vi "TrackerMain.vi"(11 "MeasureConfig":T1={"Bead locations"=[{"X"=0, "Y"=0}], "ROI"=200, "Experiment base path"=path "", "Image output subdir"="images", "Output mode"=enum."None", "Traces output subdir"="traces", "QTrk Settings"={"Image width"=150, "Image height"=150, "Number of threads (CPU based)"=-1, "CUDA Device"=-2, "COM Background correction factor"=0.0, "ZLUT MinRadius"=8.0, "ZLUT Radial sample density"=5.0, "ZLUT Angular sample density"=2.0, "ZLUT ROI Coverage"=0.7, "QI Iterations"=1, "QI MinRadius"=2.0, "QI Radial sample density"=5.0, "QI Angular sample density"=2.0, "QI ROI Coverage"=0.7, "QI Angular Step \nIteration Factor"=0.8, "XCOR Profile Length"=1, "XCOR Profile Width"=128, "XCOR Iterations"=32, "Gaussian 2D Fit Iterations"=2, "Gaussian 2D Sigma (pixels)"=3.0, "Downsample"=0}, "Tracking Config"={"Number of steps"=0, "ZLUT stepsize (um)"=0.0, "Z correction factor"=0.0, "Start piezo Z (um)"=0.0, "Pixel size (nm)"=0.0, "2D Localization Type"=enum."Quadrant Interpolation", "Z Command (None)"=enum."Nothing", "Z Piezo scale"=FALSE, "ZLUT Building\nimages per frame"=0, "ZLUT Bias correction planes"=1}, "Experiment Name"="", "Program"={"Commands"=[], "Motor Axis accuracy conditions"={"Magnet Z"=0.0, "Magnet rotation"=0.0, "Camera"={"X"=0.0, "Y"=0.0}, "Piezo XY"={"X"=0.0, "Y"=0.0}, "Piezo Z"=0.0}, "Axis flags"={"Magnet Z"=FALSE, "Magnet rotation"=FALSE, "Camera"={"X"=FALSE, "Y"=FALSE}, "Piezo XY"={"X"=FALSE, "Y"=FALSE}, "Piezo Z"=FALSE}}, "ZLUT"=[], "Camera settings"={"Framerate (Hz)"=60, "Exposure time (us)"=5000, "Image size"={"Width"=1280, "Height"=1024}, "Number of buffers"=30}, "Experiment Script"="", "Max frames in memory"=10000, "Save traces as binary"=FALSE, "Pixel Calibration Gain Image"="camera_calib_gain.bin", "Pixel Calibration Offset Image"="camera_calib_offset.bin", "Use pixel calibration images"=FALSE, "Internal camera settings"="", "Trace write interval"=100, "ExperimentComment"=""} {"QTrk Settings"."QI ROI Coverage" format="%_2g"; "QTrk Settings"."QI MinRadius" format="%.2f"; "QTrk Settings"."QI Angular sample density" format="%.3f"; "QTrk Settings"."QI Radial sample density" format="%.2f"; "QTrk Settings"."ZLUT Radial sample density" format="%.2f"; "QTrk Settings"."ZLUT MinRadius" format="%.2f"}) -> (0 "Section list":i32[](array[numeric]))   [LabVIEW 2011]
uses:
  Typedefs/MeasureConfigType.ctl
  Typedefs/MeasureConfigOutputMode.ctl
  qtrk/QTrkLVBinding/QTrkSettings.ctl
  Typedefs/TrackingConfigType.ctl
  qtrk/QTrkLVBinding/QTrkLocalizationType.ctl
  qtrk/QTrkLVBinding/QTrkZCommandType.ctl
  ExperimentProgram/ExperimentProgramType.ctl
  ExperimentProgram/ExProgCommandType.ctl
  ExperimentProgram/ExProgCommandEnumType.ctl
  Motors/MotorAxisEnum.ctl
  Motors/MotorPosType.ctl
  Typedefs/XYf.ctl
  Motors/MotorPosFlagsType.ctl
  Camera/GenericCameraConfigType.ctl
  Typedefs/CmdEnum_UserInterfaceCmd.ctl
  qtrk/QTrkLVBinding/ResultManagerConfig.ctl
  qtrk/QTrkLVBinding/XYZf.ctl
  Camera/CIGrabParams.ctl
  qtrk/QTrkLVBinding/QTrkInstance.ctl
  qtrk/QTrkLVBinding/ResultManagerInstance.ctl
  Camera/CIGrabControlMsg.ctl
  Camera/CIGrabControlMsgEnum.ctl
  GlobalVariables.vi
panel:
  out "ZLUT Correction":sgl[][](graph)
  out "Lost frames":i32
  in  "Offset factor":dbl=1.0
  in  "Gain factor":dbl=1.0
  in  "Close dialog":bool
  out "Framerate":i32
  out "Localizations done":i32
  out "Captured frames":i32
  out "Tracker internal profiling info":string
  out "Tracking queue %":i32
  out "[base]\\traces\\[expname].txt":path
  out "[base]\\traces\\[expname]_motors.txt":path
  out "Saved frames":i32
  out "Time (s)":dbl
  out "Script Complete":bool
  out "Instruction index":i32
  in  "End experiment":bool
  out "Frames complete":i32
  # "Running experiment"
  # "(used for commands with string parameters)"
  # "-2: Use all devices\n-1: Use best device"
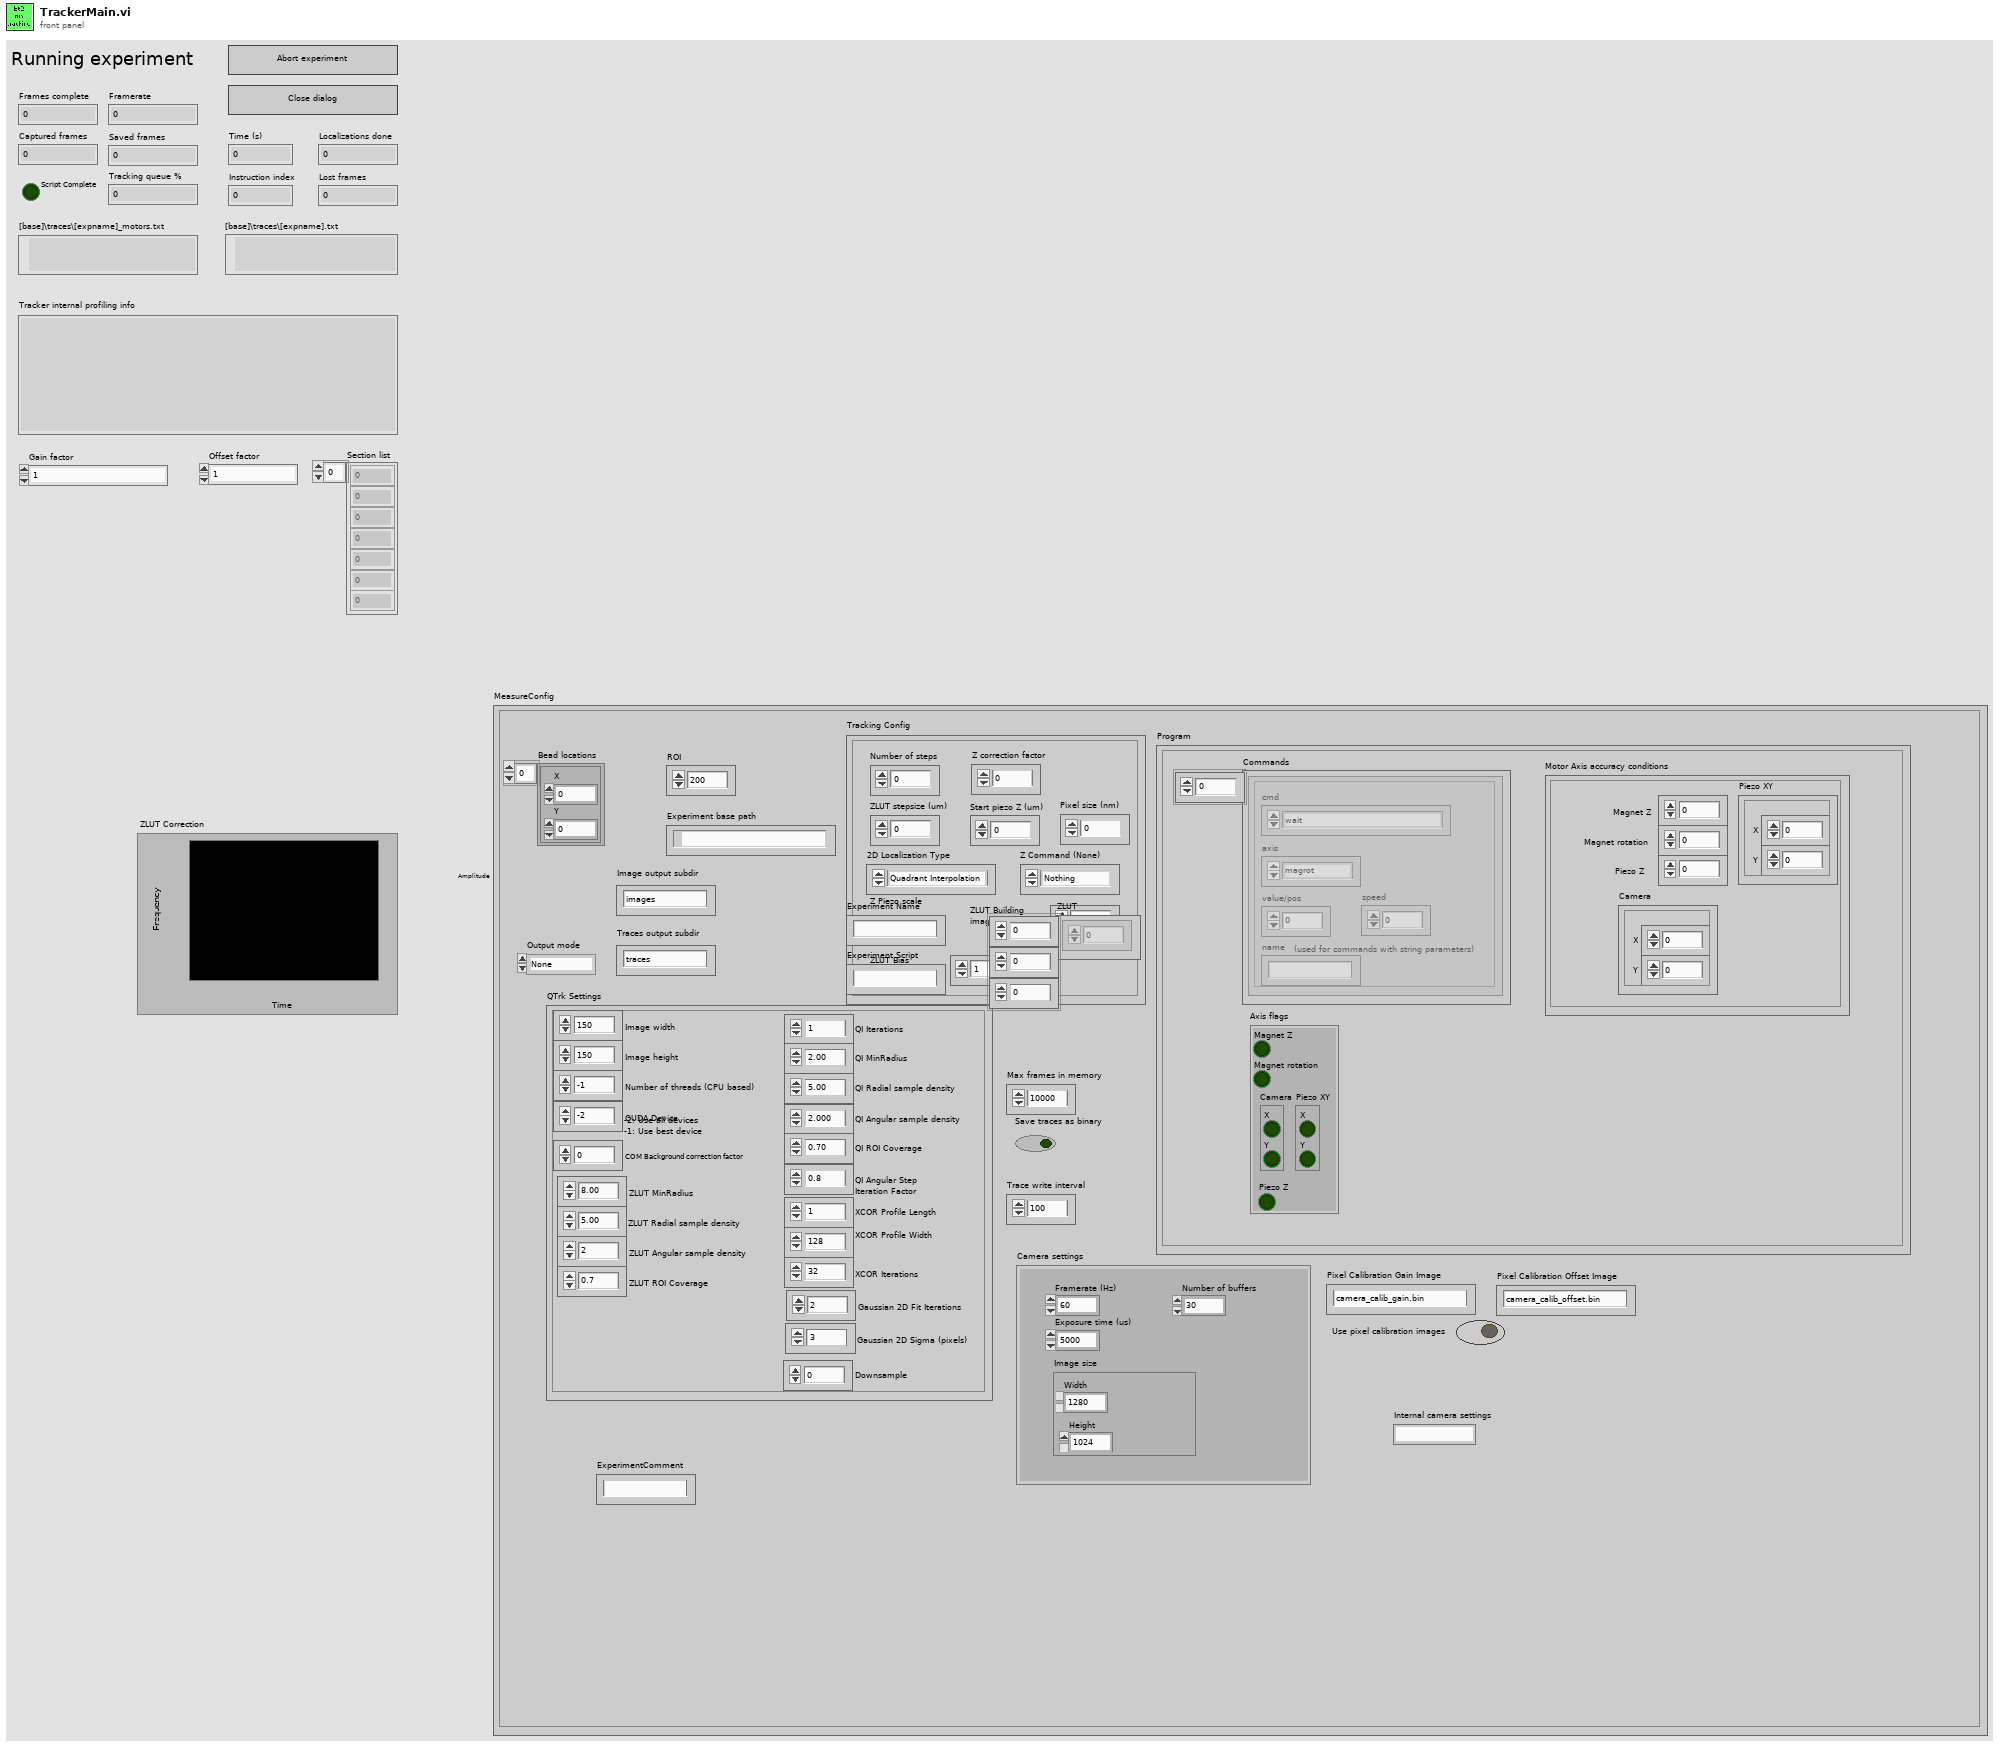
[diagram p1: front panel]
types:
  T1 = typedef "MeasureConfigType.ctl" = cluster{"Bead locations":cluster{"X":i32, "Y":i32}[], "ROI":i32, "Experiment base path":path, "Image output subdir":string, "Output mode":T2, "Traces output subdir":string, "QTrk Settings":T3, "Tracking Config":T4, "Experiment Name":string, "Program":T7, "ZLUT":sgl[][][], "Camera settings":T14, "Experiment Script":string, "Max frames in memory":i32, "Save traces as binary":bool, "Pixel Calibration Gain Image":string, "Pixel Calibration Offset Image":string, "Use pixel calibration images":bool, "Internal camera settings":string, "Trace write interval":i32, "ExperimentComment":string}
  T2 = typedef "MeasureConfigOutputMode.ctl" = enum16{"None", "Track", "SaveImages"}
  T3 = typedef "QTrkSettings.ctl" = cluster{"Image width":i32, "Image height":i32, "Number of threads (CPU based)":i32, "CUDA Device":i32, "COM Background correction factor":sgl, "ZLUT MinRadius":sgl, "ZLUT Radial sample density":sgl, "ZLUT Angular sample density":sgl, "ZLUT ROI Coverage":sgl, "QI Iterations":i32, "QI MinRadius":sgl, "QI Radial sample density":sgl, "QI Angular sample density":sgl, "QI ROI Coverage":sgl, "QI Angular Step \nIteration Factor":sgl, "XCOR Profile Length":i32, "XCOR Profile Width":i32, "XCOR Iterations":i32, "Gaussian 2D Fit Iterations":i32, "Gaussian 2D Sigma (pixels)":sgl, "Downsample":i32}
  T4 = typedef "TrackingConfigType.ctl" = cluster{"Number of steps":i32, "ZLUT stepsize (um)":sgl, "Z correction factor":sgl, "Start piezo Z (um)":sgl, "Pixel size (nm)":sgl, "2D Localization Type":T5, "Z Command (None)":T6, "Z Piezo scale":bool, "ZLUT Building\nimages per frame":i32, "ZLUT Bias correction planes":i32}
  T5 = typedef "QTrkLocalizationType.ctl" = enum16{"Center-of-Mass", "1D Cross-Correlation", "Quadrant Interpolation", "Gaussian 2D MLE", "QI + ZLUTAlign", "ZLUTAlign", "QI + FourierLUT"}
  T6 = typedef "QTrkZCommandType.ctl" = enum16{"Nothing", "ComputeZ", "BuildRadialZLUT", "BuildImageZLUT", "RadialZLUT+ImageZLUT"}
  T7 = typedef "ExperimentProgramType.ctl" = cluster{"Commands":T8[], "Motor Axis accuracy conditions":T11, "Axis flags":T13}
  T8 = typedef "ExProgCommandType.ctl" = cluster{"cmd":T9, "axis":T10, "value/pos":dbl, "speed":dbl, "name":string}
  T9 = typedef "ExProgCommandEnumType.ctl" = enum16{"wait", "move", "event", "idle", "when", "section", "stop"}
  T10 = typedef "MotorAxisEnum.ctl" = enum16{"no axis", "magrot", "magpos", "px", "py", "pz", "camx", "camy"}
  T11 = typedef "MotorPosType.ctl" = cluster{"Magnet Z":dbl, "Magnet rotation":dbl, "Camera":T12, "Piezo XY":T12, "Piezo Z":dbl}
  T12 = typedef "XYf.ctl" = cluster{"X":sgl, "Y":sgl}
  T13 = typedef "MotorPosFlagsType.ctl" = cluster{"Magnet Z":bool, "Magnet rotation":bool, "Camera":cluster{"X":bool, "Y":bool}, "Piezo XY":cluster{"X":bool, "Y":bool}, "Piezo Z":bool}
  T14 = typedef "GenericCameraConfigType.ctl" = cluster{"Framerate (Hz)":i32, "Exposure time (us)":i32, "Image size":cluster{"Width":i32, "Height":i32}, "Number of buffers":i32}
  T15 = typedef "CmdEnum_UserInterfaceCmd.ctl" = enum32{"Idle (Use for default)", "ResultTracesUpdated", "MeasureConfigUpdated", "MeasureEnd", "MeasureStart"}
  T16 = typedef "ResultManagerConfig.ctl" = cluster{"Number of beads":i32, "Number of frame info columns":i32, "Result scaling":T17, "Result offset":T17, "Write Interval":i32, "Max frames in memory":i32, "Binary output (1/0)":i8}
  T17 = typedef "XYZf.ctl" = cluster{"X":sgl, "Y":sgl, "Z":sgl}
  T18 = typedef "ResultManagerInstance.ctl" = cluster{"InstancePtr":u64}
  T19 = typedef "QTrkInstance.ctl" = cluster{"QTrk Pointer":u64}
  T20 = typedef "CIGrabParams.ctl" = cluster{"QTrk Instance":T19, "ResultManager":T18, "Send to queue?":bool, "Force full-frame capture":bool}
  T21 = typedef "CIGrabControlMsg.ctl" = cluster{"Msg":T22}
  T22 = typedef "CIGrabControlMsgEnum.ctl" = enum16{"Stop", "EnableTracking", "DisableTracking"}
  T23 = typedef "PixelCalibrationDataType.ctl" = cluster{"Offset image":T24, "Gain image":T24, "Use offset":bool, "Use gain":bool}
  T24 = typedef "IMAQ Image.ctl" = refnum<image>
  T25 = typedef "CameraInstance.ctl" = cluster{"VI refs":T26, "Camera state":variant}
  T26 = typedef "CameraInterface.ctl" = cluster{"Close":T27, "Get/Set generic config":T28, "Grab":T29, "Show Settings Dialog":T30, "AdjustBeadPos":T31, "Save/load camera settings":T32}
  T27 = typedef "CICloseType.ctl" = refnum<vi>
  T28 = typedef "CIGetSetGenericConfig.ctl" = refnum<vi>
  T29 = typedef "CIGrabType.ctl" = refnum<vi>
  T30 = typedef "CISettingsDlg.ctl" = refnum<vi>
  T31 = typedef "CIAdjustBeadPos.ctl" = refnum<vi>
  T32 = typedef "CISaveLoadSettings.ctl" = refnum<vi>
  T33 = typedef "ExProgState.ctl" = cluster{"Wanted Motorpos":T11, "Goal motorpos":T11, "Instruction":i32, "Speed":T11, "New instruction?":bool, "Instruction start time":dbl}
  T34 = typedef "QueueListType.ctl" = cluster{"Motor In":refnum<queue>, "User Interface Image View":refnum<queue>, "User Interface Camera Control":refnum<queue>, "User Interface Event Notifier":refnum<notifier>, "Initialized?":bool, "Experiment Script Event Notifier":refnum<notifier>}
  T35 = cluster{"Script loop delay":i32, "Motor loop ":i32, "Motor get pos wait time\nper axis":i32}
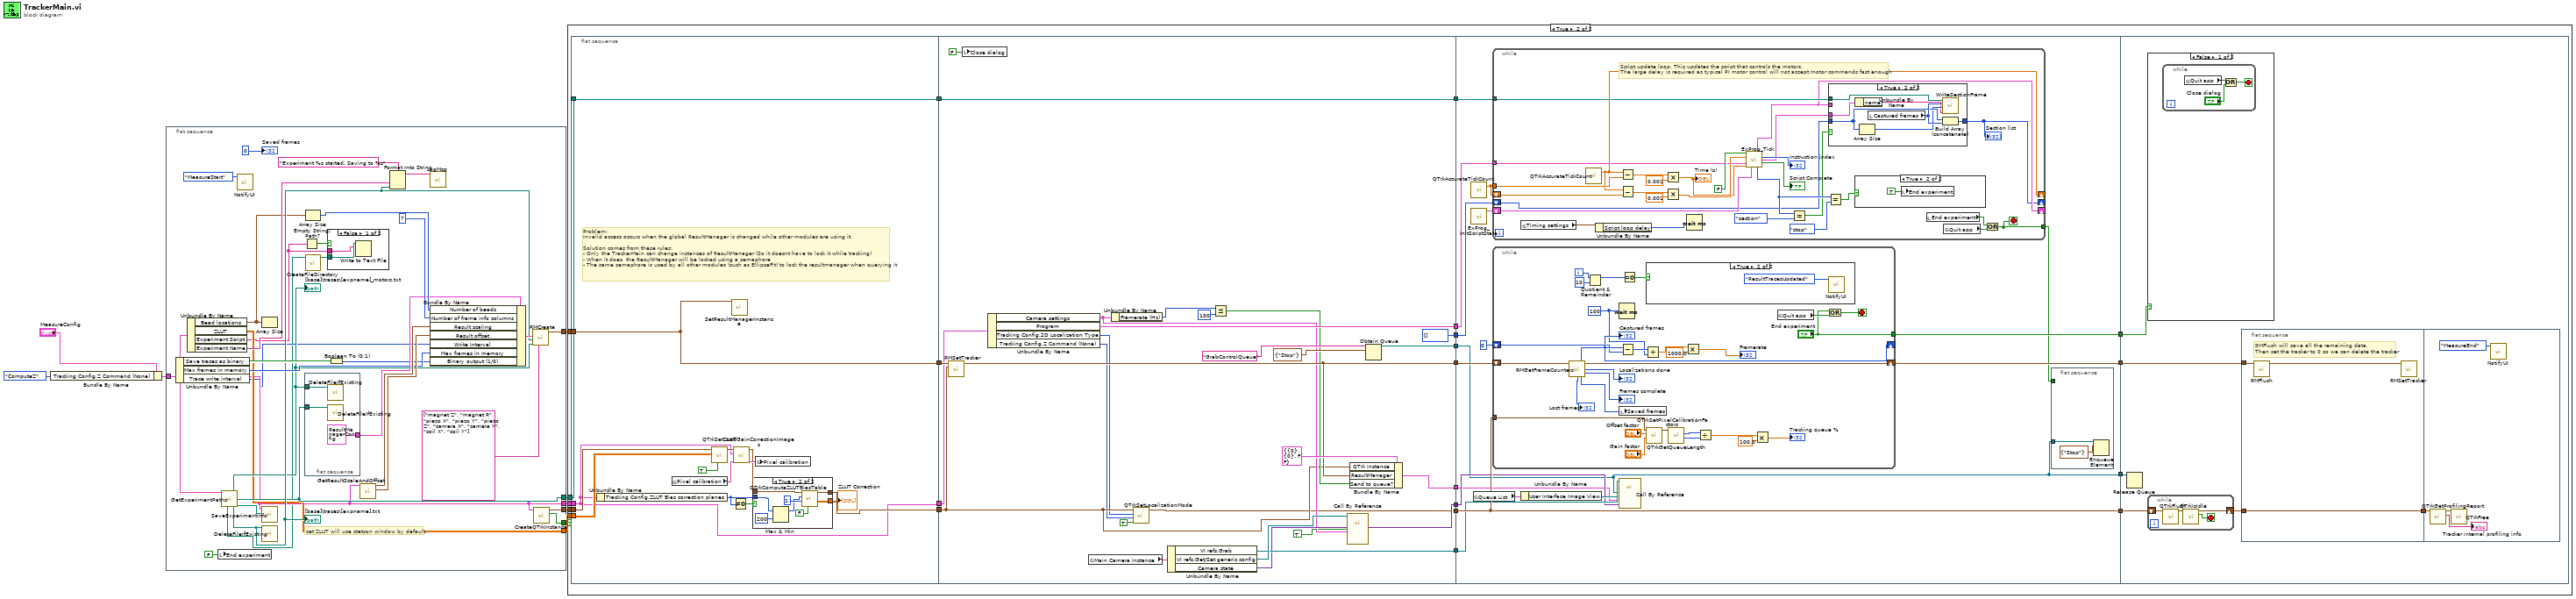
[diagram p0: block diagram]
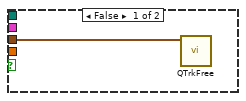
[diagram p2: hidden frame]
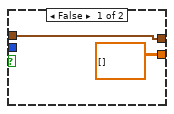
[diagram p3: hidden frame]
diagram:
  n1 = Bundle By Name(cluster="MeasureConfig", "Tracking Config.Z Command (None)"=QTrkZCommandType."ComputeZ") -> (w2:T1)
  n2 = flat-sequence {
    tunnel: [w19] -> w9
    tunnel: [w22] -> w7
    tunnel: [w21] -> w8
    tunnel: [w20] -> w6
    tunnel: [w16] -> w5
    tunnel: [w18] -> w4
    tunnel: w2 -> [w16]
    frame #0 {
      # "set ZLUT will use stetson window by default"
      n3 = Unbundle By Name(w16) -> ("Save traces as binary"=w29:bool, "Max frames in memory"=w30:i32, "Trace write interval"=w11:i32)
      n4 = Unbundle By Name(w16) -> ("Bead locations"=w17:cluster{"X":i32, "Y":i32}[], "ZLUT"=w20:sgl[][][], "Experiment Script"=w15:string, "Experiment Name"=w26:string)
      n5 = local write "End experiment"(FALSE ("End experiment")) -> ()
      n6 = call "GetExperimentPaths.vi"("MeasureConfig"=w16) -> ("[base]\\traces\\[expname]_motors.txt"=w23:path, "[base]\\traces\\[expname]_sections.txt"=w22:path, "[base]\\[expname]_script.txt"=w10:path, "[base]\\traces\\[expname].txt/bin"=w25:path, "[base]\\traces\\[expname]_info.txt"=w39:path)  [unwired: 6 in, 4 out]
      "[base]\\traces\\[expname]_motors.txt" <- w23
      "[base]\\traces\\[expname].txt" <- w25
      n7 = call "NotifyUI.vi"("User Interface Commands"=CmdEnum_UserInterfaceCmd."MeasureStart") -> ()  [unwired: 11 in]
      n8 = Array Size(array=w17) -> ()  [unwired: 1 out]
      n9 = call "SaveExperimentInfo.vi"("Filename"=w39, "MeasureConfig"=w16) -> ()  [unwired: 10 in]
      n10 = call "DeleteFileIfExisting.vi"("filename"=w25) -> ()  [unwired: 11 in]
      n11 = Empty String/Path?(string/path=w15) -> (empty?=w14:bool)
      n12 = flat-sequence {
        tunnel: [T16 {"Number of beads"=0, "Number of frame info columns"=0, "Result scaling"={"X"=0.0, "Y"=0.0, "Z"=0.0}, "Result offset"={"X"=0.0, "Y"=0.0, "Z"=0.0}, "Write Interval"=0, "Max frames in memory"=0, "Binary output (1/0)"=0} ("ResultManagerConfig")] -> w31
        tunnel: w23 -> [w44]
        tunnel: w22 -> [w43]
        frame #0 {
          n13 = call "DeleteFileIfExisting.vi"("filename"=w44) -> ()  [unwired: 11 in]
          n14 = call "DeleteFileIfExisting.vi"("filename"=w43) -> ()  [unwired: 11 in]
        }
      }
      n15 = Array Size(array=w17) -> (size(s)=w32:i32)
      n16 = call "CreateFileDirectory.vi"("filename"=w10) -> ("filename (copy)"=w38:path)  [unwired: 10 in]
      n17 = case shown="False" w14 {
        tunnel: w38 -> [w42 _]
        tunnel: w15 -> [w41 _]
        frame False {
          n18 = Write to Text File(file (use dialog)=w42, text=w41) -> ()  [unwired: 2 in, 3 out]
        }
        frame True {
        }
      }
      n19 = Boolean To (0,1)(Boolean=w29) -> (0, 1=w28:i16)
      n20 = call "GetResultScaleAndOffset.vi"("MeasureConfig"=w16) -> ("offset"=w33:cluster{dbl, dbl, "y":sgl}, "scale"=w34:cluster{sgl, sgl, sgl})  [unwired: 9 in]
      n21 = Format Into String(format string="Experiment %s started. Saving to %s", w26, w25) -> (resulting string=w24:string)  [unwired: 2 in, 1 out]
      n22 = call "LogMsg.vi"("msg"=w24) -> ()  [unwired: 11 in]
      n23 = Bundle By Name(cluster=w31, "Number of beads"=w32, "Number of frame info columns"=7, "Result scaling"=w34, "Result offset"=w33, "Write Interval"=w11, "Max frames in memory"=w30, "Binary output (1/0)"=w28) -> (w36:T16)
      n24 = call "RMCreate.vi"("Frame info names"=string[] ["magnet Z", "magnet R", "piezo X", "piezo Y", "piezo Z", "camera X", "camera Y", "coil X", "coil Y"], "frame info file"=w23, "output file"=w25, "ResultManagerConfig"=w36) -> ("ResultManager"=w21:T18)  [unwired: 7 in]
      n25 = call "CreateQTrkInstance.vi"("MeasureConfig"=w16) -> ("Go-ahead?"=w18:bool, "QTrk Instance"=w19:T19)  [unwired: 9 in]
      "Saved frames" <- 0 ("Saved frames")
    }
  }
  n26 = case shown="True" w4 {
    tunnel: w9 -> [w46 w60]
    tunnel: w8 -> [_ w59]
    tunnel: w7 -> [_ w58]
    tunnel: w6 -> [_ w57]
    tunnel: w5 -> [_ w56]
    frame False {
      n27 = call "QTrkFree.vi"("QTrk Instance"=w46) -> ()  [unwired: 6 in, 1 out]
    }
    frame True {
      n28 = flat-sequence {
        tunnel: [w79] -> w68
        tunnel: [w82] -> w67
        tunnel: w60 -> [w81]
        tunnel: w59 -> [w79]
        tunnel: w58 -> [w82]
        tunnel: w57 -> [w74]
        tunnel: w56 -> [w69]
        tunnel: [w69] -> w55
        tunnel: [w75] -> w47
        tunnel: [w115] -> w66
        tunnel: w68 -> [w119]
        tunnel: [w105] -> w65
        tunnel: [w96] -> w64
        tunnel: [i32[] [] ("initialized array")] -> w63
        tunnel: w67 -> [w117]
        tunnel: [w117] -> w62
        tunnel: [w104] -> w61
        tunnel: w55 -> [w116]
        tunnel: [w109] -> w51
        tunnel: [w107] -> w49
        tunnel: [w103] -> w48
        tunnel: w47 -> [w97]
        tunnel: w66 -> [w135]
        tunnel: w65 -> [w133]
        tunnel: w64 -> [w127]
        tunnel: w63 -> [w132]
        tunnel: w62 -> [w131]
        tunnel: w61 -> [w120]
        tunnel: [w129] -> w54
        tunnel: [w128] -> w53
        tunnel: [w127] -> w52
        tunnel: w51 -> [w126]
        tunnel: [w121] -> w50
        tunnel: w49 -> [w122]
        tunnel: w48 -> [w121]
        tunnel: w54 -> [w208]
        tunnel: w53 -> [w212]
        tunnel: w52 -> [w211]
        tunnel: w50 -> [w207]
        frame #0 {
          # "Problem: \nInvalid access occurs when the global ResultManager is changed while other modules are using it.\n\nSolution comes from these rules:\n- Only the TrackerMain can change instances of ResultManager (So it doesnt have to lock it while tracking)\n- When it does, the ResultManager will be locked using a semaphore\n- The same semaphore is used by all other modules (such as EllipseFit) to lock the resultmanager when querying it"
          n29 = Unbundle By Name(w69) -> ("Tracking Config.ZLUT Bias correction planes"=w70:i32)
          n30 = global read "GlobalVariables.vi" "Pixel calibration"() -> (w78:T23)
          n31 = call "QTrkSetZLUT.vi"("Normalize LUT"=TRUE, "ZLUT"=w74, "QTrk Instance"=w81) -> ("QTrk Instance"=w80:T19)  [unwired: 7 in, 1 out]
          n32 = call "SetResultManagerInstance.vi"("ResultManager"=w79) -> ()  [unwired: 11 in]
          n33 = Not Equal To 0?(x=w70) -> (x != 0?=w71:bool)
          n34 = call "LoadGainCorrectionImages.vi"("Pixel calibration"=w78, "MeasureConfig"=w69, "QTrk Instance in"=w80) -> ("Pixel calibration(out)"=w77:T23, "QTrk Instance out"=w76:T19)  [unwired: 7 in]
          n35 = case shown="True" w71 {
            tunnel: w76 -> [w84 w92]
            tunnel: [w84 w91] -> w75
            tunnel: [sgl[][] [] ("Bias correction table") w88] -> w73
            tunnel: w70 -> [_ w85]
            frame False {
            }
            frame True {
              n36 = Max & Min(x=w85, y=200) -> (max(x,y)=w86:i32)  [unwired: 1 out]
              n37 = call "QTrkComputeZLUTBiasTable.vi"("Use spline interpolation?"=FALSE, "smpPerPixel"=1, "bias planes"=w86, "QTrk Instance"=w92) -> ("Bias correction table"=w88:sgl[][], "QTrk Instance"=w91:T19)  [unwired: 5 in, 1 out]
            }
          }
          "ZLUT Correction" <- w73
          n38 = global write "GlobalVariables.vi" "Pixel calibration"(w77) -> ()
        }
        frame #1 {
          n39 = call "RMSetTracker.vi"("QTrk Instance"=w97, "ResultManager"=w119) -> ("ResultManager (out)"=w105:T18)  [unwired: 8 in, 1 out]
          n40 = local write "Close dialog"(FALSE ("Close dialog")) -> ()
          n41 = Unbundle By Name(w116) -> ("Camera settings"=w102:T14, "Program"=w115:T7, "Tracking Config.2D Localization Type"=w95:T5, "Tracking Config.Z Command (None)"=w94:T6)
          n42 = global read "GlobalVariables.vi" "Main Camera Instance"() -> (w111:T25)
          n43 = Unbundle By Name(w102) -> ("Framerate (Hz)"=w101:i32)
          n44 = call "QTrkSetLocalizationMode.vi"("Normalize profile"=TRUE, "Z Command"=w94, "2D Localization Type"=w95, "QTrk Instance"=w97) -> ("QTrk Instance"=w96:T19)  [unwired: 7 in]
          n45 = Unbundle By Name(w111) -> ("VI refs.Grab"=w109:T29, "VI refs.Get/Set generic config"=w110:T28, "Camera state"=w108:variant)
          n46 = Less Or Equal?(x=w101, y=100 ("x")) -> (x <= y?=w99:bool)
          n47 = call-by-ref "?"(reference=w110, "Set? (F)"=TRUE, "GenericCameraConfig"=w102, "Camera state"=w108) -> ("Camera state (out)"=w107:variant)  [unwired: 8 in, 3 out]
          n48 = Bundle By Name(cluster=T20 {"QTrk Instance"={"QTrk Pointer"=0}, "ResultManager"={"InstancePtr"=0}, "Send to queue?"=FALSE, "Force full-frame capture"=FALSE} ("TrackingParameters"), "QTrk Instance"=w97, "ResultManager"=w105, "Send to queue?"=w99) -> (w104:T20)
          n49 = Obtain Queue(name (unnamed)="GrabControlQueue", element data type=T21 {"Msg"=enum."Stop"} ("GrabControlMsg")) -> (queue out=w103:refnum<queue>)  [unwired: 3 in, 2 out]
        }
        frame #2 {
          n50 = call "QTrkAccurateTickCount.vi"() -> ("tick count (ms)"=w134:dbl)  [unwired: 2 in, 1 out]
          n51 = call "ExProg_InitScriptState.vi"() -> ("Script exec state out"=w136:T33)  [unwired: 11 in]
          n52 = global read "GlobalVariables.vi" "Queue List"() -> (w124:T34)
          n53 = while {
            shift-right: [w175] -> _
            shift-left: w136 -> [w193]
            shift-right: [w190] -> _
            shift-left: w134 -> [w194]
            tunnel: w135 -> [w174]
            tunnel: w134 -> [w189]
            shift-right: [w173] -> _
            shift-left: w132 -> [w177]
            tunnel: w131 -> [w176]
            tunnel: [w171] -> w125
            stop <- w171 stop-if-true
            # "Script update loop. This updates the script that controls the motors.\nThe large delay is required as typical PI motor control will not accept motor commands fast enough"
            n54 = global read "GlobalVariables.vi" "Timing settings"() -> (w170:T35)
            n55 = call "QTrkAccurateTickCount.vi"() -> ("tick count (ms)"=w190:dbl)  [unwired: 2 in, 1 out]
            n56 = Unbundle By Name(w170) -> ("Script loop delay"=w169:i32)
            n57 = Subtract(x=w190, y=w189) -> (x-y=w188:dbl)
            n58 = Subtract(x=w190, y=w194) -> (x-y=w185:dbl)
            n59 = Multiply(x=w188, y=0.001) -> (x*y=w183:dbl)
            "Time (s)" <- w183
            n60 = Multiply(x=w185, y=0.001) -> (x*y=w184:dbl)
            n61 = Wait (ms)(milliseconds to wait=w169) -> ()  [unwired: 1 out]
            n62 = call "ExProg_Tick.vi"("Simulation?"=FALSE, "Timestep (s)"=w184, "Program"=w174, "Current time (s)"=w183, "Script exec state in"=w193) -> ("Script exec state out"=w175:T33, "Instruction index"=→"Instruction index":i32, "Last instruction"=w172:T8, "script ended?"=→"Script Complete":bool, "Last command"=w180:T9)  [unwired: 6 in]
            n63 = Equal?(x=w180, y=ExProgCommandEnumType."section") -> (x = y?=w178:bool)
            n64 = Equal?(x=w180, y=ExProgCommandEnumType."stop") -> (x = y?=w181:bool)
            n65 = case shown="True" w178 {
              tunnel: w177 -> [w198 w202]
              tunnel: [w198 w205] -> w173
              tunnel: w176 -> [_ w204]
              tunnel: w175 -> [_ _]
              tunnel: w172 -> [_ w199]
              frame False {
              }
              frame True {
                n66 = Unbundle By Name(w199) -> ("name"=w200:string)
                n67 = Array Size(array=w202) -> (size(s)=w201:i32)
                n68 = local read "Captured frames"() -> (w203:i32)
                n69 = call "WriteSectionFrame.vi"("section name"=w200, "section index"=w201, "section frame"=w203, "[base]\\traces\\[expname]_sections.txt"=w204) -> ()  [unwired: 8 in]
                n70 = Build Array (concatenate)(w202, w203) -> (w205:i32[])
              }
            }
            "Section list" <- w173
            n71 = case shown="True" w181 {
              frame False {
              }
              frame True {
                n72 = local write "End experiment"(TRUE ("End experiment")) -> ()
              }
            }
            n73 = local read "End experiment"() -> (w197:bool)
            n74 = global read "GlobalVariables.vi" "Quit app"() -> (w196:bool)
            n75 = Or(x=w197, y=w196) -> (x .or. y?=w171:bool)
          }
          n76 = while {
            tunnel: ["End experiment"] -> w128
            tunnel: w127 -> [w143]
            shift-right: [w164] -> w129
            shift-left: w133 -> [w163]
            shift-right: [w150] -> _
            shift-left: 0 ("capturedFrames") -> [w149]
            i -> [w160]
            stop <- w166 stop-if-true
            w147 = u32 100 ("milliseconds to wait")
            n77 = call "RMGetFrameCounters.vi"("ResultManager"=w163) -> ("capturedFrames"=w150:i32, "ResultManager (out)"=w164:T18, "totalLocalizationsDone"=→"Localizations done":i32, "endFrame"=→"Frames complete":i32, "lostFrames"=→"Lost frames":i32, "lastSaveFrame"=w161:i32)  [unwired: 7 in, 2 out]
            "Captured frames" <- w150
            n78 = Quotient & Remainder(x=w160, y=10) -> (x-y*floor(x/y)=w158:i32)  [unwired: 1 out]
            n79 = Wait (ms)(milliseconds to wait=w147) -> ()  [unwired: 1 out]
            n80 = local write "Saved frames"(w161) -> ()
            n81 = Subtract(x=w150, y=w149) -> (x-y=w148:i32)
            n82 = Equal To 0?(x=w158) -> (x = 0?=w157:bool)
            n83 = Divide(x=w148, y=w147) -> (x/y=w146:dbl)
            n84 = case shown="True" w157 {
              frame False {
              }
              frame True {
                n85 = call "NotifyUI.vi"("User Interface Commands"=CmdEnum_UserInterfaceCmd."ResultTracesUpdated") -> ()  [unwired: 11 in]
              }
            }
            n86 = call "QTrkSetPixelCalibrationFactors.vi"("gainFactor (1)"="Gain factor", "offsetFactor (1)"="Offset factor", "QTrk Instance"=w143) -> ("QTrk Instance"=w140:T19)  [unwired: 7 in, 1 out]
            n87 = call "QTrkGetQueueLength.vi"("QTrk Instance"=w140) -> ("maxQueueLen"=w155:i32, "queue size"=w156:i32)  [unwired: 7 in, 2 out]
            n88 = Multiply(x=w146, y=1000.0) -> (x*y=→"Framerate":dbl)
            n89 = Divide(x=w156, y=w155) -> (x/y=w154:dbl)
            n90 = Multiply(x=w154, y=100.0) -> (x*y=→"Tracking queue %":dbl)
            n91 = global read "GlobalVariables.vi" "Quit app"() -> (w167:bool)
            n92 = Or(x="End experiment", y=w167) -> (x .or. y?=w166:bool)
          }
          n93 = Unbundle By Name(w124) -> ("User Interface Image View"=w123:refnum<queue>)
          n94 = call-by-ref "?"(reference=w126, "Camera data"=w122, "TrackingParameters"=w120, "Output Queue"=w123, "GrabControlQueue"=w121) -> ()  [unwired: 8 in, 3 out]
          n95 = flat-sequence {
            tunnel: w125 -> [_]
            tunnel: w121 -> [w138]
            frame #0 {
              n96 = Enqueue Element(queue=w138, element=T21 {"Msg"=enum."Stop"}) -> ()  [unwired: 2 in, 3 out]
            }
          }
        }
        frame #3 {
          n97 = Release Queue(queue=w207) -> ()  [unwired: 2 in, 3 out]
          n98 = case shown="False" w212 {
            frame False {
              n99 = while {
                stop <- w224 stop-if-true
                n100 = global read "GlobalVariables.vi" "Quit app"() -> (w226:bool)
                n101 = Or(x=w226, y="Close dialog") -> (x .or. y?=w224:bool)
              }
            }
            frame True {
            }
          }
          n102 = while {
            shift-right: [w223] -> w209
            shift-left: w211 -> [w221]
            stop <- w222 stop-if-true
            n103 = call "QTrkFlush.vi"("QTrk Instance"=w221) -> ("QTrk Instance (out)"=w220:T19)  [unwired: 9 in, 1 out]
            n104 = call "QTrkIsIdle.vi"("QTrk Instance"=w220) -> ("Currently idle?"=w222:bool, "QTrk Instance (out)"=w223:T19)  [unwired: 8 in, 1 out]
          }
          n105 = flat-sequence {
            tunnel: [w214] -> w210
            tunnel: w209 -> [w214]
            tunnel: w208 -> [w213]
            tunnel: w210 -> [w216]
            frame #0 {
              # "RMFlush will save all the remaining data.\nThen set the tracker to 0 so we can delete the tracker"
              n106 = call "RMFlush.vi"("ResultManager"=w213) -> ("ResultManager (out)"=w215:T18)  [unwired: 9 in, 1 out]
              n107 = call "RMSetTracker.vi"("ResultManager"=w215) -> ()  [unwired: 9 in, 2 out]
            }
            frame #1 {
              n108 = call "QTrkGetProfilingReport.vi"("QTrk Instance"=w216) -> ("report"=→"Tracker internal profiling info":string, "QTrk Instance (out)"=w219:T19)  [unwired: 9 in]
              n109 = call "QTrkFree.vi"("QTrk Instance"=w219) -> ()  [unwired: 6 in, 1 out]
              n110 = call "NotifyUI.vi"("User Interface Commands"=CmdEnum_UserInterfaceCmd."MeasureEnd") -> ()  [unwired: 11 in]
            }
          }
        }
      }
    }
  }
